vi "Shoulder Angle to Target Wrist Angle.vi"(8 "Target Wrist Angle (-1,1)":dbl(knob) scale=-1.0..1.0, 10 "Shoulder angle deg(0-180)":dbl) -> (2 "Target Wrist angle deg(90-270)":dbl)   [LabVIEW 2023]
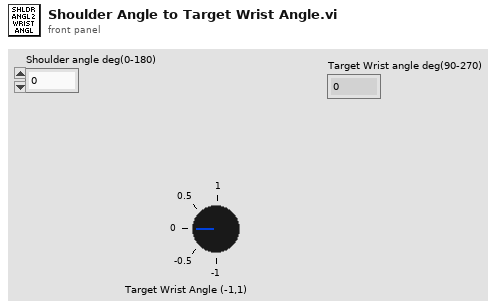
[diagram p1: front panel]
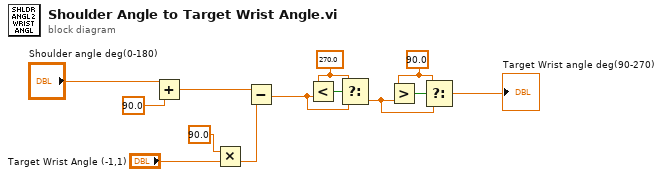
[diagram p0: block diagram]
diagram:
  w8 = 90.0 ("x")
  w10 = 270.0 ("t")
  n1 = Add(x="Shoulder angle deg(0-180)", y=90.0) -> (x+y=w5:dbl)
  n2 = Multiply(x=90.0, y="Target Wrist Angle (-1,1)") -> (x*y=w2:dbl)
  n3 = Subtract(x=w5, y=w2) -> (x-y=w4:dbl)
  n4 = Less?(x=w10, y=w4) -> (x < y?=w11:bool)
  n5 = Select(t=w10, s=w11, f=w4) -> (s? t:f=w7:dbl)
  n6 = Greater?(x=w8, y=w7) -> (0:w9:bool)
  n7 = Select(t=w8, s=w9, f=w7) -> (s? t:f=→"Target Wrist angle deg(90-270)":dbl)
